vi "DriveExecute.vi"(8 "error in (no error)":errorcluster) -> (0 "error out":errorcluster)   [LabVIEW 2023]
doc: "Execute for Drie\n\nClosed control loop for drive\n\ninput: \n error in (cluster)\n\noutput:\n error out (cluster)"
uses:
  <vilib>/Rock Robotics/WPI/ThirdParty/JAS_Junk/TrajLib/LinearFilter_ResetToValue.vi
  <vilib>/Rock Robotics/WPI/ThirdParty/JAS_Junk/TrajLib/LinearFilter_Calculate.vi
  DriveGlobal.vi
  <vilib>/Rock Robotics/WPI/ThirdParty/JAS_Junk/TrajLib/LinearFilter_MovingAverage.vi
  <vilib>/Rock Robotics/WPI/ThirdParty/JAS_Junk/TrajLib/LinearFilter_LowPassBW1.vi
  <vilib>/Rock Robotics/WPI/ThirdParty/JAS_Junk/TrajLib/LinearFilter_LowPassBW2.vi
  <vilib>/Rock Robotics/WPI/ThirdParty/JAS_Junk/TrajLib/LinearFilter_HighPassBW1.vi
  <vilib>/Rock Robotics/WPI/ThirdParty/JAS_Junk/TrajLib/LinearFilter_HighPassBW2.vi
  <vilib>/Rock Robotics/WPI/ThirdParty/JAS_Junk/TrajLib/Trajectory_Library.lvlib
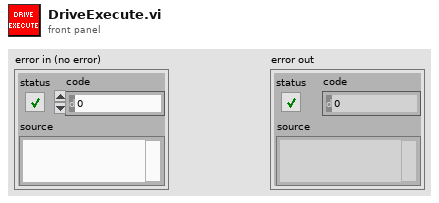
[diagram p1: front panel]
types:
  T1 = enum16{"Moving Average", "Low Pass 1st Order Butterworth", "Low Pass 2nd Order Butterworth", "High Pass 1st Order Butterworth", "High Pass 2nd Order Butterworth"}
  T2 = typedef "Trajectory_Library.lvlib/CHASSIS_SPEEDS.ctl" = cluster{"vX":dbl, "vY":dbl, "vOmega":dbl}
  T3 = typedef "ADIS16470 Device Reference.ctl" = cluster{"DevStatus":errorcluster, "Hardware Config":T4, "Calibration Complete":refnum<notifier>, "Status Reference":refnum<data-value>, "Data Reference":refnum<data-value>, "Sychronous Process VI":T8, "Cmd FIFO":refnum<k33>, "Source":T9, "Data FIFO":refnum<k33>, "Calibration Time (ms)":u32, "Data Reference":refnum<data-value>}
  T4 = typedef "ADIS16470 Hardware Configuration.ctl" = cluster{"SPI Clock Rate (Hz)":dbl, "IMU SPI Mode (3)":T5, "IMU Reset Pin":T6, "IMU SPI Bus":T7, "IMU Data Ready Pin":T6, "Stall Config":cluster{"Pow2BytesPerRead":u8, "StallTicks":u16, "CsToSclkTicks":u8}}
  T5 = typedef "WPI_SPIMode.ctl" = enum16{"Mode 0 (Clk Idle Low,Sample on Leading)", "Mode 1 (Clk Idle Low,Sample on Trailing)", "Mode 2 (Clk Idle High,Sample on Leading)", "Mode 3 (Clk Idle High,Sample on Trailing)"}
  T6 = typedef "FPGA_DIOChannel.ctl" = enum8{"DIO 0", "DIO 1", "DIO 2", "DIO 3", "DIO 4", "DIO 5", "DIO 6", "DIO 7", "DIO 8", "DIO 9", "DIO MXP 0", "DIO MXP 1", "DIO MXP 2", "DIO MXP 3", "DIO MXP 4", "DIO MXP 5", "DIO MXP 6", "DIO MXP 7", "DIO MXP 8", "DIO MXP 9", "DIO MXP 10", "DIO MXP 11", "DIO MXP 12", "DIO MXP 13", "DIO MXP 14", "DIO MXP 15", "SPI Port CS1", "SPI Port CS2", "SPI Port CS3", "SPI Port MISO", "SPI Port MOSI", "Invalid"}
  T7 = typedef "spi_bus.ctl" = enum16{"SPI On-Board, CS0", "SPI On-Board, CS1", "SPI On-Board, CS2", "SPI On-Board, CS3", "SPI MXP", "Invalid"}
  T8 = typedef "ADIS16470 Process.ctl" = refnum<vi>
  T9 = typedef "FPGA_CounterEncoderSourceConvertionLVSourceType.ctl" = cluster{"DevStatus":errorcluster, "AnalogTriggerMode?":bool, "DigitalMode":cluster{"DIO Channel":T10}, "AnalogTriggerMode":cluster{"AnalogTriggerIndex":T11, "OutputType":T12}}
  T10 = typedef "FPGA_DIODigitalSourceChannel.ctl" = enum8{"DIO 0", "DIO 1", "DIO 2", "DIO 3", "DIO 4", "DIO 5", "DIO 6", "DIO 7", "DIO 8", "DIO 9", "DIO MXP 0", "DIO MXP 1", "DIO MXP 2", "DIO MXP 3", "DIO MXP 4", "DIO MXP 5", "DIO MXP 6", "DIO MXP 7", "DIO MXP 8", "DIO MXP 9", "DIO MXP 10", "DIO MXP 11", "DIO MXP 12", "DIO MXP 13", "DIO MXP 14", "DIO MXP 15", "SPI Port CS1", "SPI Port CS2", "SPI Port CS3", "SPI Port MISO", "SPI Port MOSI", "Disabled"}
  T11 = typedef "FPGA_AnalogTriggerIndex.ctl" = enum8{"Trig 0", "Trig 1", "Trig 2", "Trig 3", "Trig 4", "Trig 5", "Trig 6", "Trig 7", "Invalid"}
  T12 = typedef "FPGA_AnalogTriggerOutType.ctl" = enum16{"InWindow", "TriggerState", "Rising", "Falling"}
  T13 = typedef "Trajectory_Library.lvlib/SWERVE_DRIVE_KINEMATICS.ctl" = cluster{"NumModules":i32, "InverseKinematics":T14, "ForwardKinematics":T14, "Modules":T15[], "PrevCoR":T15, "SavedModuleStates":T16[]}
  T14 = typedef "NI_Matrix.lvlib/RealMatrix.ctl" = dbl[][]
  T15 = typedef "Trajectory_Library.lvlib/TRANSLATION2D.ctl" = cluster{"X":dbl, "Y":dbl}
  T16 = typedef "Trajectory_Library.lvlib/SWERVE_DRIVE_MODULE_STATE.ctl" = cluster{"Speed":dbl, "Angle":T17}
  T17 = typedef "Trajectory_Library.lvlib/ROTATION2D.ctl" = cluster{"VALUE":dbl, "COS":dbl, "SIN":dbl}
  T18 = typedef "Trajectory_Library.lvlib/SWERVE_DRIVE_MODULE_POSITION.ctl" = cluster{"Distance":dbl, "Angle":T17, "P":bool}
  T19 = typedef "ADIS16470 Data.ctl" = cluster{"XAngle":dbl, "YAngle":dbl, "ZAngle":dbl}
  T20 = typedef "ADIS16470 Status.ctl" = cluster{"Calibrated?":bool, "IMU Detected?":bool}
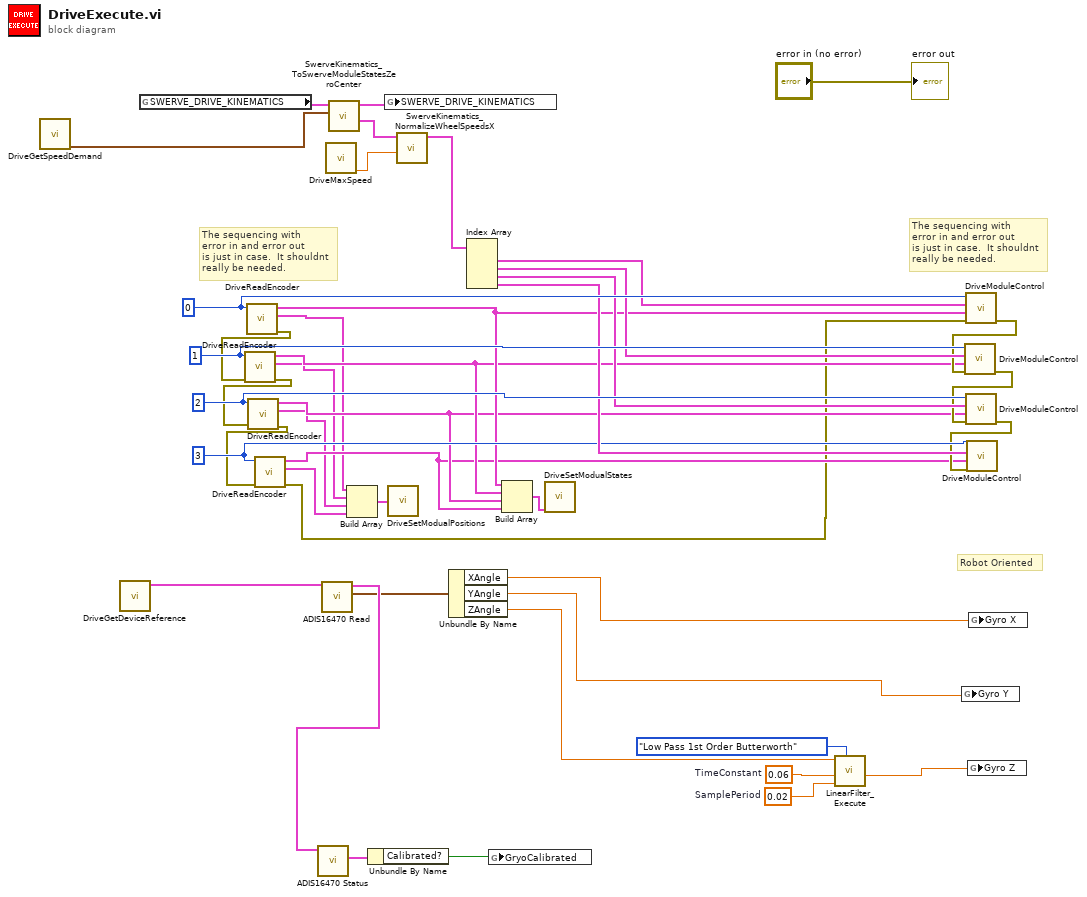
[diagram p0: block diagram]
diagram:
  w16 = 0.02  # SamplePeriod
  w15 = 0.06  # TimeConstant
  w40 = 0 ("ModualNamePrefix")
  w39 = 1 ("ModualNamePrefix")
  w38 = 2 ("ModualNamePrefix")
  w33 = 3 ("ModualNamePrefix")
  # "Robot Oriented"
  # "The sequencing with\nerror in and error out\nis just in case.  It shouldnt\nreally be needed."
  # "The sequencing with\nerror in and error out\nis just in case.  It shouldnt\nreally be needed."
  n1 = call "DriveGetSpeedDemand.vi"() -> ("ChassisSpeedDemand"=w42:T2)  [unwired: 8 in, 3 out]
  n2 = call "DriveGetDeviceReference.vi"() -> ("ADIS16470DevRef out"=w13:T3)  [unwired: 11 in]
  n3 = global read "DriveGlobal.vi" "SWERVE_DRIVE_KINEMATICS"() -> (w43:T13)
  n4 = call "DriveReadEncoder.vi"("ModualNamePrefix"=w40) -> ("error out"=w19:errorcluster, "SWERVE_DRIVE_MODULE_POSITION"=w25:T18, "SWERVE_DRIVE_MODULE_STATE"=w29:T16)  [unwired: 8 in]
  n5 = call "DriveReadEncoder.vi"("error in"=w19, "ModualNamePrefix"=w39) -> ("error out"=w18:errorcluster, "SWERVE_DRIVE_MODULE_POSITION"=w24:T18, "SWERVE_DRIVE_MODULE_STATE"=w28:T16)  [unwired: 7 in]
  n6 = call "DriveReadEncoder.vi"("error in"=w18, "ModualNamePrefix"=w38) -> ("error out"=w17:errorcluster, "SWERVE_DRIVE_MODULE_POSITION"=w23:T18, "SWERVE_DRIVE_MODULE_STATE"=w27:T16)  [unwired: 7 in]
  n7 = call "DriveReadEncoder.vi"("error in"=w17, "ModualNamePrefix"=w33) -> ("error out"=w4:errorcluster, "SWERVE_DRIVE_MODULE_POSITION"=w22:T18, "SWERVE_DRIVE_MODULE_STATE"=w26:T16)  [unwired: 7 in]
  n8 = call <vilib>:"ADIS16470 Read.vi"("ADIS16470DevRef"=w13) -> ("ADIS16470 Value"=w9:T19, "ADIS16470DevRef"=w10:T3)  [unwired: 7 in, 2 out]
  n9 = call <vilib>:"ADIS16470 Status.vi"("ADIS16470DevRef"=w10) -> ("ADIS16470 Status"=w12:T20)  [unwired: 8 in, 2 out]
  n10 = call "DriveMaxSpeed.vi"() -> ("Max Speed (m/sec)"=w2:dbl)  [unwired: 10 in, 1 out]
  n11 = call <vilib>:"SwerveKinematics_ToSwerveModuleStatesZeroCenter.vi"("ChassisSpeeds"=w42, "in SWERVE_DRIVE_KINEMATICS"=w43) -> ("ModuleStates"=w3:T16[], "out SWERVE_DRIVE_KINEMATICS"=w41:T13)  [unwired: 8 in]
  n12 = Build Array(w25, w24, w23, w22) -> (w20:T18[])
  n13 = Unbundle By Name(w12) -> ("Calibrated?"=w11:bool)
  n14 = global write "DriveGlobal.vi" "SWERVE_DRIVE_KINEMATICS"(w41) -> ()
  n15 = call "DriveSetModualPositions.vi"("Swerve_Drive_Modual_Position"=w20) -> ()  [unwired: 11 in]
  n16 = call <vilib>:"SwerveKinematics_NormalizeWheelSpeedsX.vi"("AttainableMaxSpeed"=w2, "in WheelStates"=w3) -> ("out WheelStates"=w1:T16[])  [unwired: 9 in]
  n17 = Unbundle By Name(w9) -> ("XAngle"=w7:dbl, "YAngle"=w6:dbl, "ZAngle"=w8:dbl)
  n18 = Index Array(array=w1) -> (element #1=w34:T16, element #2=w37:T16, element #3=w36:T16, element #4=w35:T16)  [unwired: 4 in]
  n19 = global write "DriveGlobal.vi" "GryoCalibrated"(w11) -> ()
  n20 = Build Array(w29, w28, w27, w26) -> (w21:T16[])
  n21 = call "DriveSetModualStates.vi"("Swerve__Drive_Modual_States"=w21) -> ()  [unwired: 11 in]
  n22 = call <vilib>:"LinearFilter_Execute.vi"("Filter Type"=T1."Low Pass 1st Order Butterworth", "SamplePeriod"=w16, "TimeConstant"=w15, "Input"=w8) -> ("Output"=w5:dbl)  [unwired: 6 in, 1 out]
  n23 = global write "DriveGlobal.vi" "Gyro Y"(w6) -> ()
  n24 = call "DriveModuleControl.vi"("error in"=w4, "Actual State"=w29, "Desired State"=w34, "ModualNamePrefix"=w40) -> ("error out"=w32:errorcluster)  [unwired: 7 in]
  n25 = call "DriveModuleControl.vi"("error in"=w32, "Actual State"=w28, "Desired State"=w37, "ModualNamePrefix"=w39) -> ("error out"=w31:errorcluster)  [unwired: 7 in]
  n26 = call "DriveModuleControl.vi"("error in"=w31, "Actual State"=w27, "Desired State"=w36, "ModualNamePrefix"=w38) -> ("error out"=w30:errorcluster)  [unwired: 7 in]
  n27 = call "DriveModuleControl.vi"("error in"=w30, "Actual State"=w26, "Desired State"=w35, "ModualNamePrefix"=w33) -> ()  [unwired: 7 in, 1 out]
  n28 = global write "DriveGlobal.vi" "Gyro Z"(w5) -> ()
  n29 = global write "DriveGlobal.vi" "Gyro X"(w7) -> ()
  "error out" <- "error in (no error)"
